vi "test-trapezoid-profile-ALL.vi"(8 "error in (no error)":errorcluster) -> (0 "error out":errorcluster, 3 "All TEsts passed":bool)   [LabVIEW 2019]
panel:
  out "Test 11":bool
  out "Test 10":bool
  out "Test 9":bool
  out "Test 8":bool
  out "Test 7":bool
  out "Test 6":bool
  out "Test 5":bool
  out "Test 4":bool
  out "Test 3":bool
  out "Test 2":bool
  out "Test 1":bool
  out "Test 0":bool
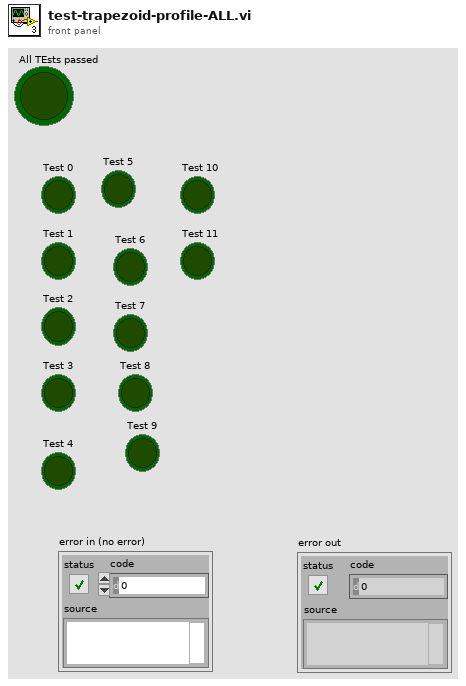
[diagram p1: front panel]
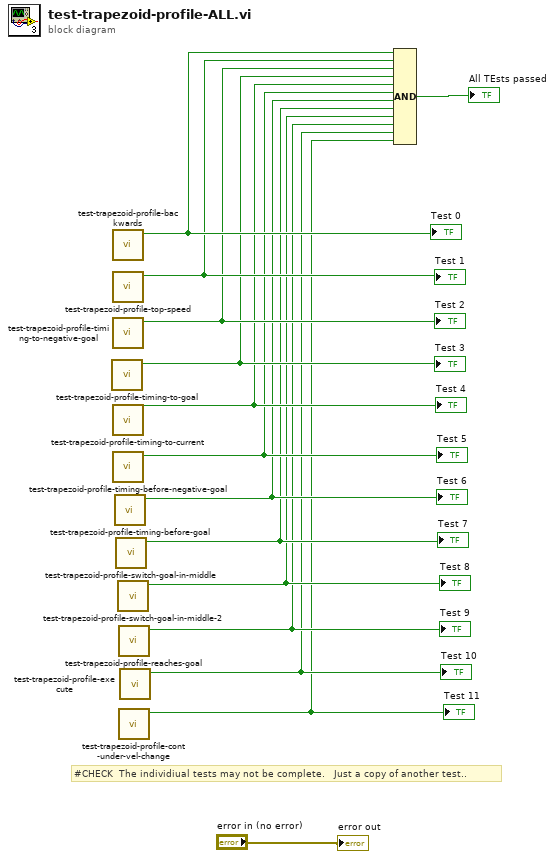
[diagram p0: block diagram]
diagram:
  # "#CHECK  The individiual tests may not be complete.   Just a copy of another test.."
  n1 = call "test-trapezoid-profile-timing-to-goal.vi"() -> ("Test Passed"=w10:bool)  [unwired: 11 in]
  "Test 3" <- w10
  n2 = call "test-trapezoid-profile-backwards.vi"() -> ("Test Passed"=w13:bool)  [unwired: 11 in]
  "Test 0" <- w13
  n3 = call "test-trapezoid-profile-top-speed.vi"() -> ("Test Passed"=w12:bool)  [unwired: 11 in]
  "Test 1" <- w12
  n4 = call "test-trapezoid-profile-timing-to-negative-goal.vi"() -> ("Test Passed"=w11:bool)  [unwired: 11 in]
  "Test 2" <- w11
  n5 = call "test-trapezoid-profile-timing-to-current.vi"() -> ("Test Passed"=w9:bool)  [unwired: 11 in]
  "Test 4" <- w9
  n6 = call "test-trapezoid-profile-timing-before-negative-goal.vi"() -> ("Test Passed"=w8:bool)  [unwired: 11 in]
  "Test 5" <- w8
  n7 = call "test-trapezoid-profile-timing-before-goal.vi"() -> ("Test Passed"=w7:bool)  [unwired: 11 in]
  "Test 6" <- w7
  n8 = call "test-trapezoid-profile-switch-goal-in-middle.vi"() -> ("Test Passed"=w6:bool)  [unwired: 11 in]
  "Test 7" <- w6
  n9 = call "test-trapezoid-profile-switch-goal-in-middle-2.vi"() -> ("Test Passed"=w5:bool)  [unwired: 11 in]
  "Test 8" <- w5
  n10 = call "test-trapezoid-profile-reaches-goal.vi"() -> ("Test Passed"=w4:bool)  [unwired: 11 in]
  "Test 9" <- w4
  n11 = call "test-trapezoid-profile-cont-under-vel-change.vi"() -> ("Test Passed"=w2:bool)  [unwired: 11 in]
  "Test 11" <- w2
  n12 = call "test-trapezoid-profile-execute.vi"() -> ("Test Passed"=w3:bool)  [unwired: 11 in]
  "Test 10" <- w3
  n13 = Compound Arithmetic op=AND(w13, w12, w11, w10, w9, w8, w7, w6, w5, w4, w3, w2) -> (→"All TEsts passed":bool)
  "error out" <- "error in (no error)"
